vi "Class - Inheritance Parent Libraries.vi"(7 "Msg Chain":string, 8 "error in (no error)":errorcluster {"code" format="Error %.0f"}, 10 "Classes":refnum<class "Class Documentation.lvclass">[](array[class]), 11 "VIDoc Printer - Confluence In":refnum<class "VIDoc Printer - Confluence.lvclass">) -> (0 "error out":errorcluster {"code" format="Error %.0f"}, 3 "VIDoc Printer - Confluence Out":refnum<class "VIDoc Printer - Confluence.lvclass">)   [LabVIEW 2023, in "VIDoc Printer - Confluence.lvlib" / "VIDoc Printer - Confluence.lvclass"]
uses:
  VIDoc Printer - Confluence.lvclass
  C:/projects/DMC/Tooling/Git-Action-Service/Source/Documentation Generation/Printers/Printer/VIDoc Printer.lvclass
  Parsing/Class Documentation/Class Documentation.lvclass
  Parsing/Class Documentation/Class Documentation.lvclass/Class Documentation.ctl
  Confluence Formatting/Types/Format Combo Box.ctl
  Settings/Printer Settings/Detail Level Enum.ctl
  Parsing/Class Documentation/Get Owning Library Info.vi
  Parsing/Class Documentation/Get Name.vi
  VIDoc Printer - Confluence.lvclass/VIDoc Printer - Confluence.ctl
  Printer/VIDoc Printer.lvclass
  UI Interaction/UI Interaction.lvclass
  Confluence Formatting/Confluence Formatting.lvlib
  Settings/Printer Settings/Printer Settings.lvclass
  C:/projects/DMC/Tooling/Git-Action-Service/Source/Documentation Generation/Printers/Confluence Printer/VIDoc Printer - Confluence.lvclass
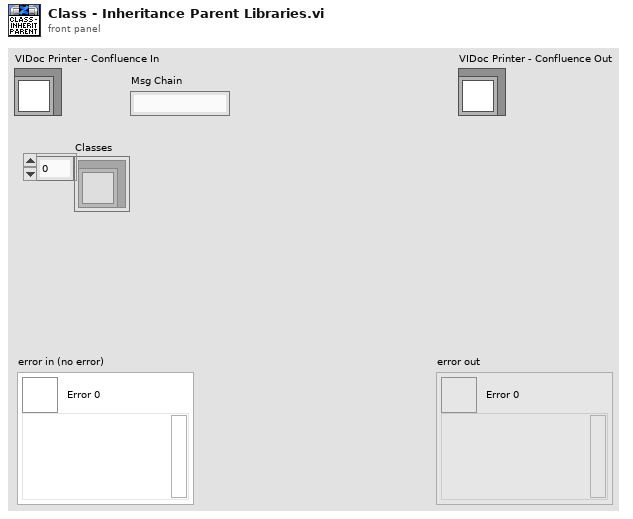
[diagram p1: front panel]
types:
  T1 = typedef "VIDoc Printer.lvlib/Printer Settings.lvclass/Detail Level Enum.ctl" = enum16{"None", "Minimal", "Standard", "Full"}
  T2 = typedef "Confluence Formatting.lvlib/Format Combo Box.ctl" = string
  T3 = typedef "VIDoc Parsing.lvlib/Base Library Info Cluster.ctl" = cluster{"Name":string, "Icon":T4, "Version":cluster{"Major":u16, "Minor":u16, "Fix":u16, "Build":u16}, "Description":string, "Path":path, "Friends":string[], "Library Scope":enum32{"invalid scope", "public", "private", "protected", "community"}, "Qualified Name":string}
  T4 = typedef "imagedata.ctl" = cluster{"image type":i32, "image depth":i32, "image":u8[], "mask":u8[], "colors":u32[], "Rectangle":cluster{"left":i16, "top":i16, "right":i16, "bottom":i16}}
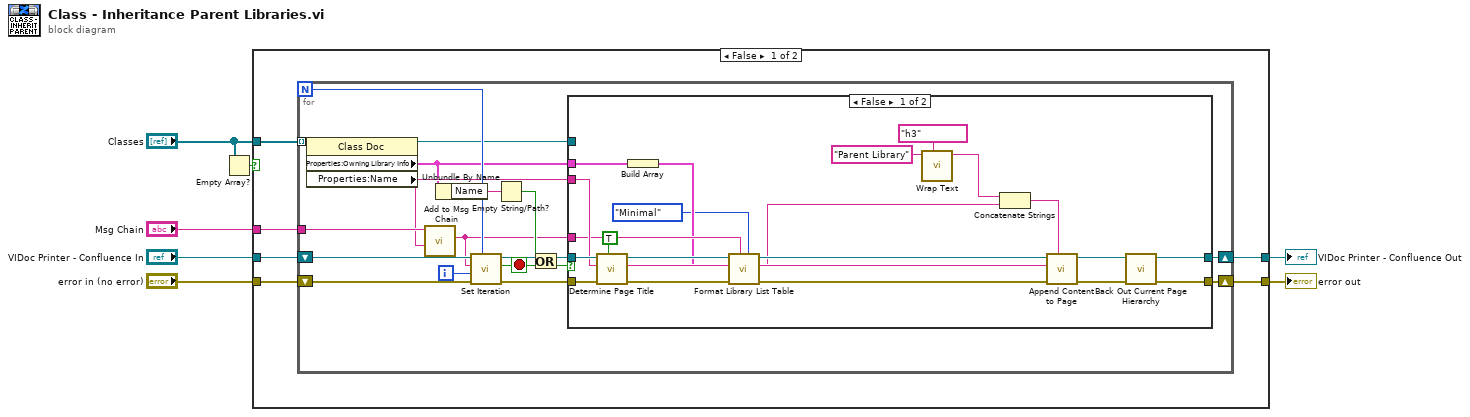
[diagram p0: block diagram]
diagram:
  n1 = Empty Array?(array="Classes") -> (empty?=w7:bool)
  n2 = case shown="False" w7 {
    tunnel: [w13 w56] -> w2
    tunnel: [w12 w57] -> w1
    tunnel: "error in (no error)" -> [w11 w56]
    tunnel: "Classes" -> [w10 _]
    tunnel: "VIDoc Printer - Confluence In" -> [w9 w57]
    tunnel: "Msg Chain" -> [w8 _]
    frame False {
      n3 = for {
        N -> [w24]
        shift-right: [w29] -> w13
        shift-left: w11 -> [w27]
        shift-right: [w30] -> w12
        shift-left: w9 -> [w28]
        tunnel: w10 -> [w31] mode=indexing
        tunnel: w8 -> [w22]
        i -> [w23]
        stop <- w19 stop-if-true
        n4 = property class="Class Doc"(reference=w31) -> (reference out=w20:refnum<class "Class Documentation.lvclass">, "Properties:Owning Library Info"=w18:T3, "Properties:Name"=w21:string)  [unwired: 1 in, 1 out]
        n5 = call "Add to Msg Chain.vi"("New"=w21, "Msg Chain in"=w22) -> ("Msg Chain out"=w14:string)  [unwired: 9 in]
        n6 = Unbundle By Name(w18) -> ("Name"=w17:string)
        n7 = call "Set Iteration.vi"("Progress Max"=w24, "error in (no error)"=w27, "Progress Value"=w23, "Message (No Message Update)"=w14, "VIDoc Printer In"=w28) -> ("error out"=w25:errorcluster, "Abort?"=w19:bool, "VIDoc Printer Out"=w26:refnum<class "VIDoc Printer - Confluence.lvclass">)  [unwired: 4 in]
        n8 = Empty String/Path?(string/path=w17) -> (empty?=w15:bool)
        n9 = Or(x=w15, y=w19) -> (x .or. y?=w16:bool)
        n10 = case shown="False" w16 {
          tunnel: [w41 w54] -> w30
          tunnel: [w43 w55] -> w29
          tunnel: w18 -> [w35 _]
          tunnel: w26 -> [w50 w54]
          tunnel: w25 -> [w49 w55]
          tunnel: w21 -> [w48 _]
          tunnel: w20 -> [_ _]
          tunnel: w14 -> [w36 _]
          frame False {
            n11 = call "Determine Page Title.vi"("Update Current Page (F)"=TRUE, "error in (no error)"=w49, "Name"=w48, "VIDoc Printer - Confluence In"=w50) -> ("error out"=w38:errorcluster, "Page Title"=w53:string, "VIDoc Printer - Confluence Out"=w40:refnum<class "VIDoc Printer - Confluence.lvclass">)  [unwired: 4 in, 1 out]
            n12 = Build Array(w35) -> (w34:T3[])
            n13 = call "Format Library List Table.vi"("Detail Level"=Detail_Level_Enum."Minimal", "Msg Chain in"=w36, "error in (no error)"=w38, "Library Info Array"=w34, "VIDoc Printer - Confluence In"=w40) -> ("error out"=w37:errorcluster, "Table Text"=w32:string, "VIDoc Printer - Confluence Out"=w39:refnum<class "VIDoc Printer - Confluence.lvclass">)  [unwired: 4 in]
            n14 = call "Wrap Text.vi"("Formatting"=T2 "h3", "String"="Parent Library") -> ("Wrapped String"=w46:string)  [unwired: 8 in, 1 out]
            n15 = Concatenate Strings(w46, w32) -> (w45:string)
            n16 = call "Append Content to Page.vi"("Page Content"=w45, "error in (no error)"=w37, "Page Title"=w53, "VIDoc Printer - Confluence In"=w39) -> ("error out"=w52:errorcluster, "VIDoc Printer - Confluence Out"=w42:refnum<class "VIDoc Printer - Confluence.lvclass">)  [unwired: 6 in]
            n17 = call "Back Out Current Page Hierarchy.vi"("error in (no error)"=w52, "VIDoc Printer - Confluence In"=w42) -> ("error out"=w43:errorcluster, "VIDoc Printer - Confluence Out"=w41:refnum<class "VIDoc Printer - Confluence.lvclass">)  [unwired: 8 in]
          }
          frame True {
          }
        }
      }
    }
    frame True {
    }
  }
  "error out" <- w2
  "VIDoc Printer - Confluence Out" <- w1
